vi "Create IUnregisteredHandler.vi"(8 "error in (no error)":errorcluster, 11 "IWampMessage":refnum<class "IWampMessage.lvclass">) -> (0 "error out":errorcluster, 3 "IUnregisteredHandler out":refnum<class "IUnregisteredHandler.lvclass">)   [LabVIEW 2020, in "wamplv.lvlib"]
uses:
  wamplv.lvlib
  SerialisedMessages/JSONMessage/WampMessage JSON.lvclass
  SerialisedMessages/MsgPackMessage/WampMessage MsgPack.lvclass
  SerialisedMessages/IWampMessage/IWampMessage.lvclass
  UnregisteredHandler/UnregisteredHandler.lvclass
  UnregisteredHandler MsgPack/UnregisteredHandler MsgPack.lvclass
  C:/local/wamplv/Private/Requests/IGenericInternalMessage/IGenericInternalMessage.lvclass
  C:/local/wamplv/Private/Requests/IInternalMessage/IInternalMessage.lvclass
  C:/local/wamplv/Private/Requests/MessageReceivedHandlers/Unregistered/IUnregisteredHandler.lvclass
  C:/local/wamplv/Private/Requests/MessageReceivedHandlers/Unregistered/UnregisteredHandler/UnregisteredHandler.lvclass
  C:/local/wamplv/Private/Requests/MessageReceivedHandlers/IJsonMessageHandler/IJsonMessageHandler.lvclass
  C:/local/wamplv/Private/Requests/MessageReceivedHandlers/Unregistered/UnregisteredHandler MsgPack/UnregisteredHandler MsgPack.lvclass
  C:/local/wamplv/Private/Requests/MessageReceivedHandlers/IMsgPackMessageHandler/IMsgPackMessageHandler.lvclass
  IUnregisteredHandler.lvclass
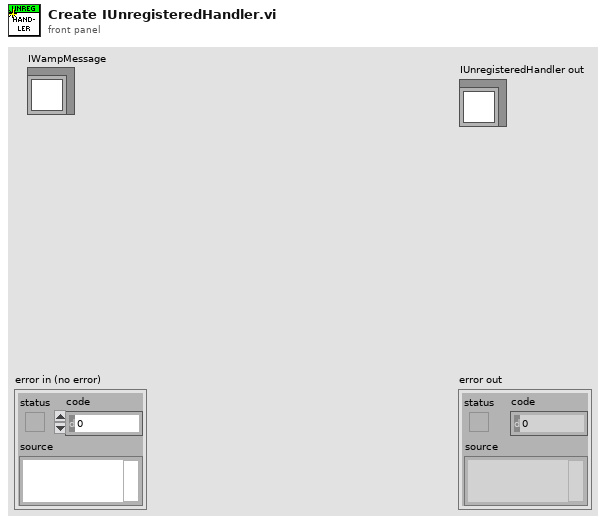
[diagram p1: front panel]
types:
  T1 = typedef "wamplv.lvlib/WAMP Client.lvclass/Serialisation.ctl" = enum16{"JSON", "MessagePack"}
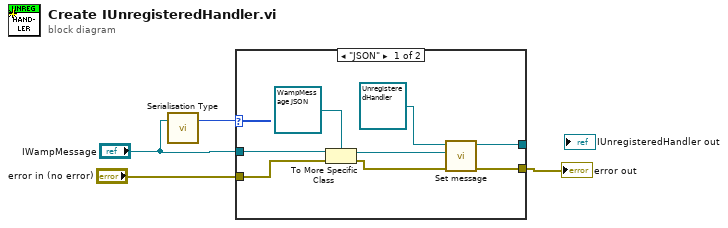
[diagram p0: block diagram]
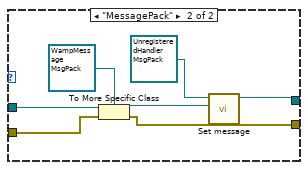
[diagram p2: hidden frame]
diagram:
  n1 = call-dynamic "Serialisation Type.vi"("IWampMessage in"="IWampMessage") -> ("Serialisation Type"=w4:T1)  [unwired: 2 in]
  n2 = case shown="\"JSON\"" w4 {
    tunnel: "IWampMessage" -> [w11 w18]
    tunnel: "error in (no error)" -> [w9 w17]
    tunnel: [w7 w14] -> _
    tunnel: [w5 w12] -> w1
    frame "JSON" {
      n3 = To More Specific Class(target class=refnum<class "WampMessage JSON.lvclass"> refnum ("wamplv.lvlib:JSONMessage.lvclass"), reference=w11, error in=w9) -> (specific class reference=w6:refnum<class "WampMessage JSON.lvclass">, error out=w5:errorcluster)
      n4 = call-dynamic "Set message.vi"("WampMessage JSON"=w6, "IMsgPackMessageHandler in"=refnum<class "UnregisteredHandler.lvclass"> refnum ("wamplv.lvlib:UnregisteredHandler.lvclass")) -> ("IMsgPackMessageHandler out"=w7:refnum<class "UnregisteredHandler.lvclass">)  [unwired: 9 in]
    }
    frame "MessagePack" {
      n5 = To More Specific Class(target class=refnum<class "WampMessage MsgPack.lvclass"> refnum ("wamplv.lvlib:MsgPackMessage.lvclass"), reference=w18, error in=w17) -> (specific class reference=w13:refnum<class "WampMessage MsgPack.lvclass">, error out=w12:errorcluster)
      n6 = call-dynamic "Set message.vi"("WampMessage MsgPack"=w13, "UnregisteredHandler MsgPack in"=refnum<class "UnregisteredHandler MsgPack.lvclass"> refnum ("wamplv.lvlib:UnregisteredHandler MsgPack.lvclass")) -> ("UnregisteredHandler MsgPack out"=w14:refnum<class "UnregisteredHandler MsgPack.lvclass">)  [unwired: 9 in]
    }
  }
  "error out" <- w1
